vi "merge orbit and crossing info.vi"(10 "crossing stats":T3={"recent crossing"=93287.088128, "prev crossing"=93285.965824, "crossing-2"=93284.859904, "number of crossings"=20040, "period"=2.2282240000058664, "new crossing"=FALSE, "new odd crossing"=FALSE, "slope"=0.0}, 11 "orbit parameters":T2) -> (3 "orbit parameters with crossing":T1)   [LabVIEW 2017]
uses:
  typedefs/crossing stats.ctl
  typedefs/orbit parameters full.ctl
  typedefs/orbit parameters with crossing info.ctl
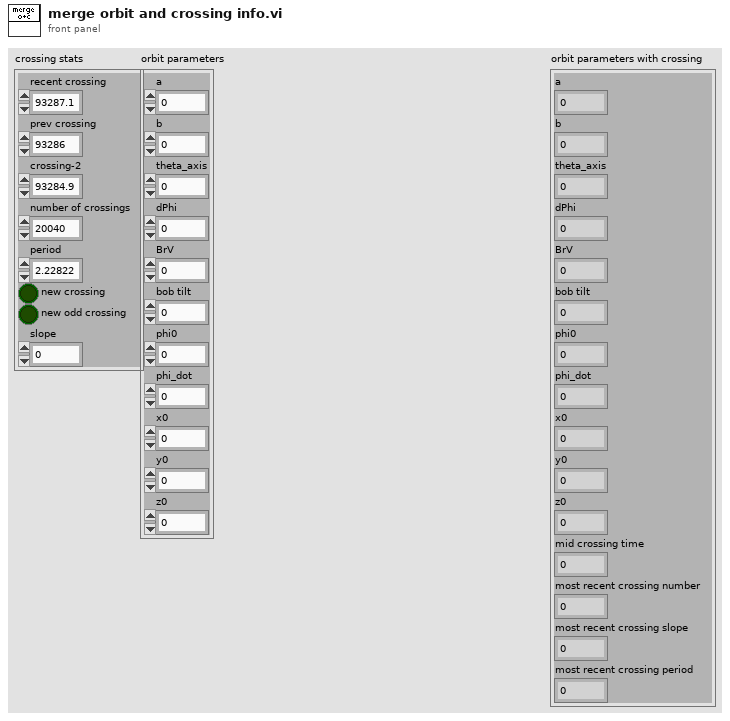
[diagram p1: front panel]
types:
  T1 = typedef "orbit parameters with crossing info.ctl" = cluster{"a":dbl, "b":dbl, "theta_axis":dbl, "dPhi":dbl, "BrV":dbl, "bob tilt":dbl, "phi0":dbl, "phi_dot":dbl, "x0":dbl, "y0":dbl, "z0":dbl, "mid crossing time":dbl, "most recent crossing number":dbl, "most recent crossing slope":dbl, "most recent crossing period":dbl}
  T2 = typedef "orbit parameters full.ctl" = cluster{"a":dbl, "b":dbl, "theta_axis":dbl, "dPhi":dbl, "BrV":dbl, "bob tilt":dbl, "phi0":dbl, "phi_dot":dbl, "x0":dbl, "y0":dbl, "z0":dbl}
  T3 = typedef "crossing stats.ctl" = cluster{"recent crossing":dbl, "prev crossing":dbl, "crossing-2":dbl, "number of crossings":i32, "period":dbl, "new crossing":bool, "new odd crossing":bool, "slope":dbl}
  T4 = cluster{"[0]":dbl, "[1]":dbl, "[2]":dbl, "[3]":dbl, "[4]":dbl, "[5]":dbl, "[6]":dbl, "[7]":dbl, "[8]":dbl, "[9]":dbl, "[10]":dbl, "[11]":dbl, "[12]":dbl, "[13]":dbl, "[14]":dbl}
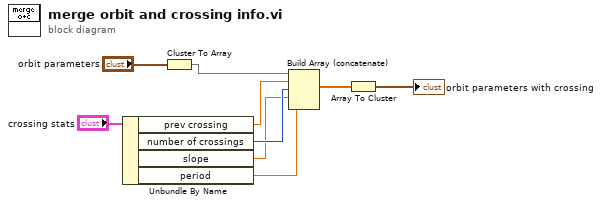
[diagram p0: block diagram]
diagram:
  n1 = Unbundle By Name("crossing stats") -> ("prev crossing"=w6:dbl, "number of crossings"=w5:i32, "slope"=w4:dbl, "period"=w3:dbl)
  n2 = Cluster To Array(cluster="orbit parameters") -> (array=w7:dbl[])
  n3 = Build Array (concatenate)(w7, w6, w5, w4, w3) -> (w2:dbl[])
  n4 = Array To Cluster(array=w2) -> (cluster=→"orbit parameters with crossing":T4)
